vi "Move or Stop Range Target.vi"(8 "error in (no error)":errorcluster, 10 "Target Speed & Direction":i16=128, 11 "Range Controller Actor in":refnum<class "Range Controller Actor.lvclass">) -> (0 "error out":errorcluster, 3 "Range Controller Actor out":refnum<class "Range Controller Actor.lvclass">)   [LabVIEW 2018, in "Range Controller.lvlib" / "Range Controller Actor.lvclass"]
uses:
  Range Controller Actor.lvclass
  Range Controller Actor.lvclass/Range Controller Actor.ctl
  Reference Range Actor/Reference Range Actor Messages/Set Output State Msg/Set Output State Msg.lvclass/Set Output State Msg.ctl
  <vilib>/ActorFramework/Message Enqueuer/Message Enqueuer.lvclass/Message Enqueuer.ctl
  <vilib>/ActorFramework/Message Enqueuer/Enqueue.vi
  Reference Range Actor/Reference Range Actor Messages/Set Output State Msg/Set Output State Msg.lvclass
  C:/Program Files (x86)/National Instruments/LabVIEW 2018/vi.lib/ActorFramework/Message/Message.lvclass
  <vilib>/ActorFramework/Message Priority Queue/Priority Enqueue.vi
panel:
  # "128 is Full Stop\n0 is Full Forward\n255 is Full Reverse"
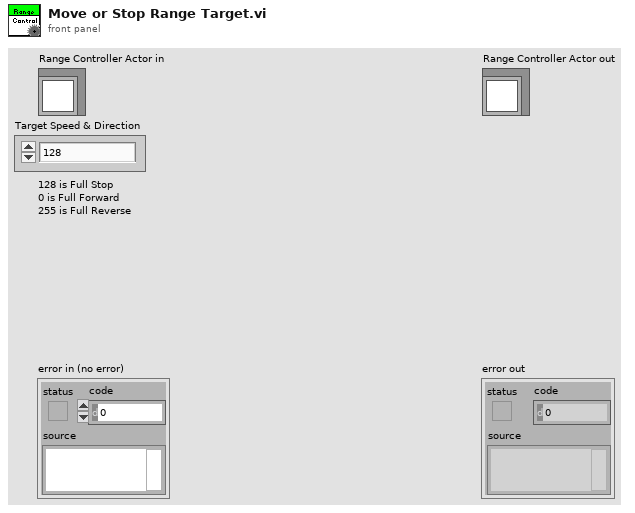
[diagram p1: front panel]
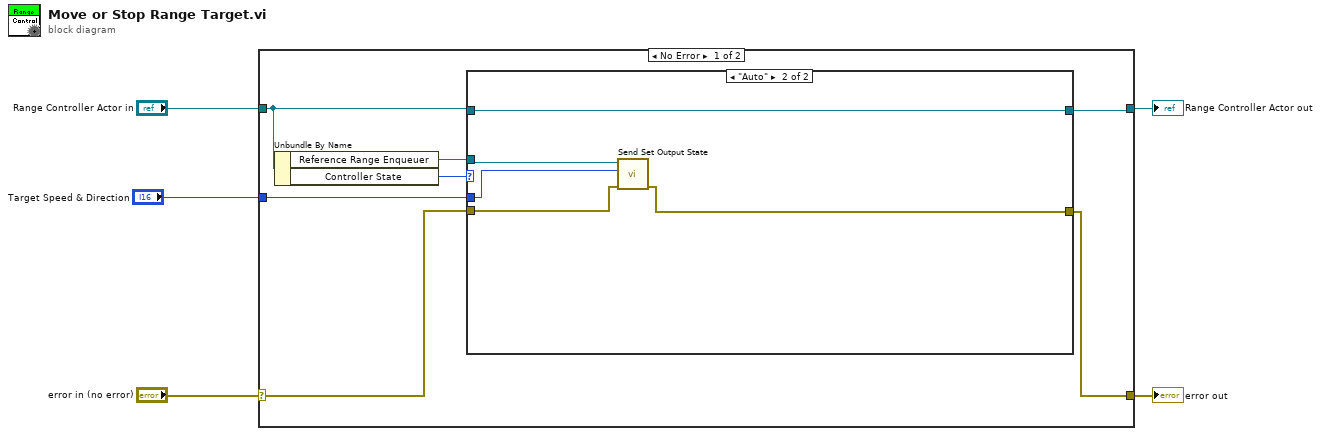
[diagram p0: block diagram]
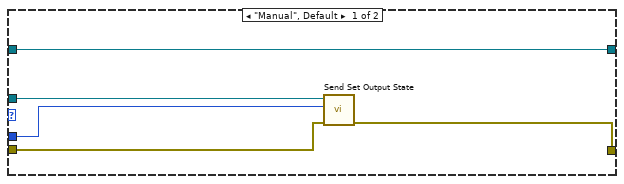
[diagram p2: hidden frame]
diagram:
  n1 = case shown="No Error" "error in (no error)" {
    selector: "error in (no error)" -> [w7 w24]
    tunnel: [w6 w24] -> w4
    tunnel: [w10 w23] -> w2
    tunnel: "Range Controller Actor in" -> [w11 w23]
    tunnel: "Target Speed & Direction" -> [w9 _]
    frame No Error {
      n2 = Unbundle By Name(w11) -> ("Reference Range Enqueuer"=w8:refnum<class "Message Enqueuer.lvclass">, "Controller State"=w12:enum16{"Manual", "Auto"})
      n3 = case shown="\"Auto\"" w12 {
        tunnel: w11 -> [w17 w22]
        tunnel: [w17 w22] -> w10
        tunnel: w9 -> [w16 w20]
        tunnel: w8 -> [w15 w21]
        tunnel: w7 -> [w14 w19]
        tunnel: [w13 w18] -> w6
        frame "Manual", Default {
          n4 = call "Send Set Output State.vi"("error in (no error)"=w14, "Speed & Direction"=w16, "Message Enqueuer in"=w15) -> ("error out"=w13:errorcluster)  [unwired: 7 in, 1 out]
        }
        frame "Auto" {
          n5 = call "Send Set Output State.vi"("error in (no error)"=w19, "Speed & Direction"=w20, "Message Enqueuer in"=w21) -> ("error out"=w18:errorcluster)  [unwired: 7 in, 1 out]
        }
      }
    }
    frame Error {
    }
  }
  "error out" <- w4
  "Range Controller Actor out" <- w2
